vi "check_moving.vi"(8 "error in (no error)":errorcluster caption="错误输入（无错误）", 10 "用户事件":refnum<user-event>, 11 "MotorSystem 输入":refnum<class "MotorSystem.lvclass">) -> (0 "error out":errorcluster caption="错误输出", 3 "MotorSystem 输出":refnum<class "MotorSystem.lvclass">)   [LabVIEW 2016, in "MotionControl_UFO_3DOF.lvlib" / "MotorSystem.lvclass"]
uses:
  <userlib>/MotionControl_UFO_3DOF/MotorSystem/MotorSystem.lvclass
  <userlib>/MotionControl_UFO_3DOF/MotorSystem/MotorSystem.lvclass/MotorSystem.ctl
  <userlib>/MotionControl_UFO_3DOF/OneMotion/OneMotion.lvclass/OneMotion.ctl
  <userlib>/MotionControl_UFO_3DOF/StepMotor/StepMotor.lvclass/StepMotor.ctl
  <userlib>/UISimCanFunc_wrapper/ctl/Notice ID.ctl
  <userlib>/MotionControl_UFO_3DOF/StepMotor/StepMotor.lvclass
  <userlib>/MotionControl_UFO_3DOF/OneMotion/OneMotion.lvclass
  <userlib>/UISimCanFunc_wrapper/UISimCanFunc_wrapper.lvlib
panel:
  out "moving?":bool[](array[boolean])
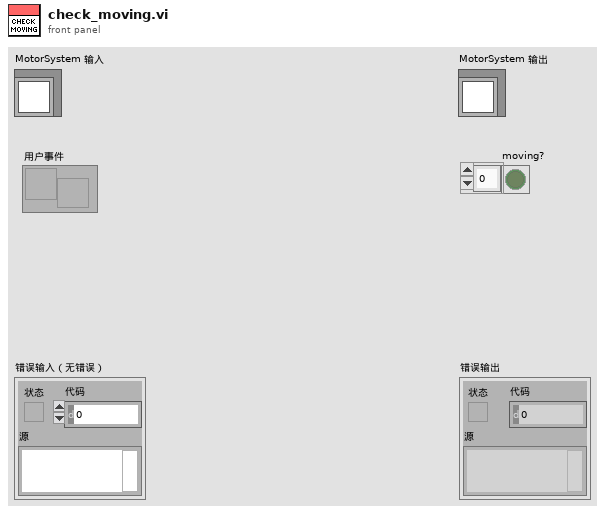
[diagram p1: front panel]
types:
  T1 = typedef "UISimCanFunc_wrapper.lvlib/Notice ID.ctl" = enum16{"S1 FALLING", "S1 RISING", "S2 FALLING", "S2 RISING", "S3 FALLING", "S3 RISING", "P4 DOUT LOW", "P4 DOUT HIGH", "MOVE DONE (OPEN LOOP)", "MOVE DONE (CLOSED LOOP)", "ORIGIN ARRIVED", "STALL NOTIFY", "MOVING", "STANDBY", "SET_TARGET_POS", "OTHERS"}
  T2 = typedef "MotionControl_UFO_3DOF.lvlib/MotorSystem.lvclass/MotionCluster.ctl" = cluster{"OneMotion.lvclass":refnum<class "OneMotion.lvclass">, "connected?":bool, "default enabled?":bool, "enabled?":bool}
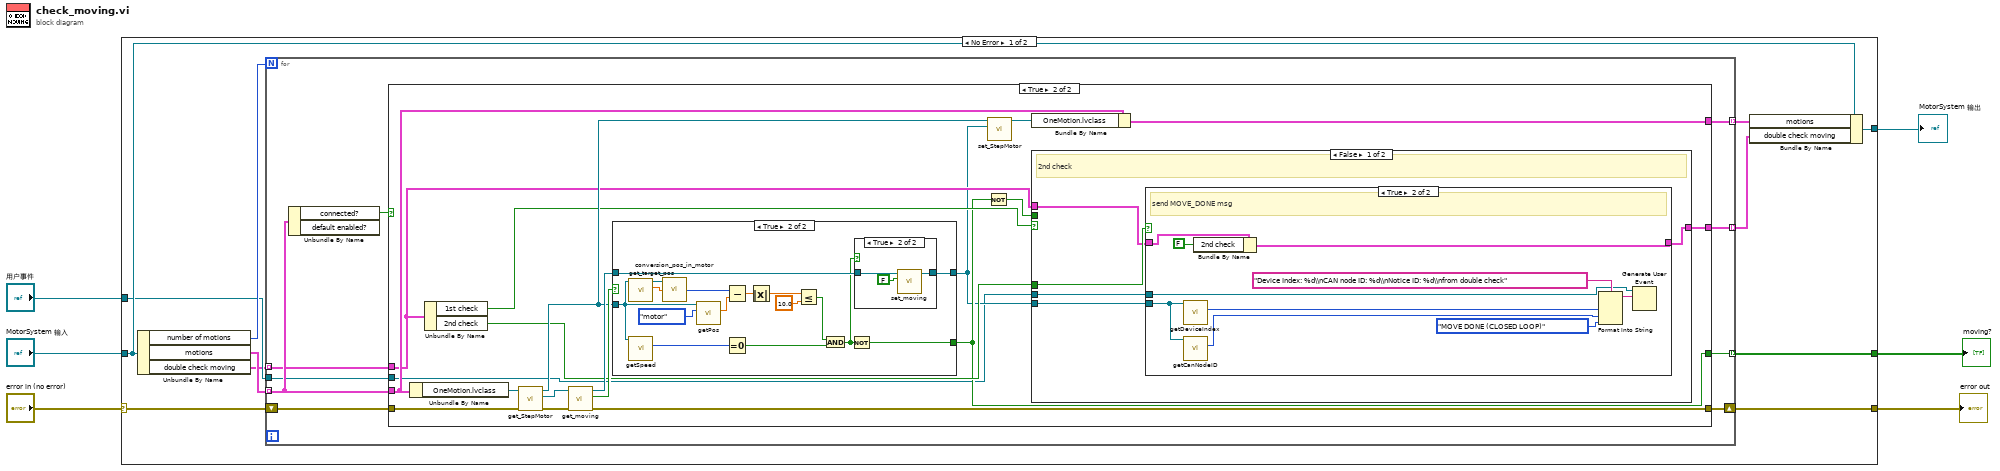
[diagram p0: block diagram]
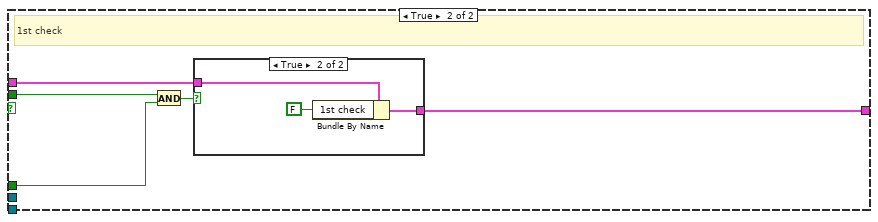
[diagram p4: hidden frame]
diagram:
  n1 = case shown="No Error" "error in (no error)" {
    tunnel: [w17 _] -> w4
    tunnel: "MotorSystem 输入" -> [w11 w96]
    tunnel: [w16 _] -> w3
    tunnel: [w13 w96] -> w5
    tunnel: "用户事件" -> [w10 _]
    selector: "error in (no error)" -> [w7 _]
    frame No Error {
      n2 = Unbundle By Name(w11) -> ("number of motions"=w15:i32, "motions"=w12:T2[], "double check moving"=w9:cluster{"1st check":bool, "2nd check":bool}[])
      n3 = for {
        N: w15 -> [_]
        tunnel: [w25] -> w16 mode=indexing
        tunnel: w12 -> [w23] mode=indexing
        shift-right: [w26] -> w17
        shift-left: w7 -> [w24]
        tunnel: [w21] -> w14 mode=indexing
        tunnel: w10 -> [w20]
        tunnel: w9 -> [w19] mode=indexing
        tunnel: [w18] -> w8 mode=indexing
        n4 = Unbundle By Name(w23) -> ("connected?"=w22:bool)  [unwired: 1 out]
        n5 = case shown="True" w22 {
          tunnel: [w29 w45] -> w26
          tunnel: [_ w34] -> w25
          tunnel: w23 -> [w28 w40]
          tunnel: w24 -> [w29 w44]
          tunnel: [w28 w38] -> w21
          tunnel: w20 -> [_ w30]
          tunnel: w19 -> [w27 w33]
          tunnel: [w27 w32] -> w18
          frame False {
          }
          frame True {
            n6 = Unbundle By Name(w40) -> ("OneMotion.lvclass"=w48:refnum<class "OneMotion.lvclass">)
            n7 = Unbundle By Name(w33) -> ("1st check"=w37:bool, "2nd check"=w35:bool)
            n8 = call <userlib>:"get_StepMotor.vi"("error in (no error)"=w44, "OneMotion输入"=w48) -> ("error out"=w46:errorcluster, "StepMotor.lvclass"=w47:refnum<class "StepMotor.lvclass">, "OneMotion输出"=w41:refnum<class "OneMotion.lvclass">)  [unwired: 7 in]
            n9 = call <userlib>:"get_moving.vi"("error in (no error)"=w46, "StepMotor输入"=w47) -> ("error out"=w45:errorcluster, "moving?"=w43:bool, "StepMotor输出"=w42:refnum<class "StepMotor.lvclass">)  [unwired: 7 in]
            n10 = case shown="True" w43 {
              selector: w43 -> [w74 _]
              tunnel: w41 -> [_ w81]
              tunnel: w42 -> [w75 w83]
              tunnel: [w75 w82] -> w31
              tunnel: [w74 w79] -> w34
              frame False {
              }
              frame True {
                n11 = call <userlib>:"get_target_pos.vi"("OneMotion输入"=w81) -> ("target pos"=w78:dbl, "OneMotion输出"=w91:refnum<class "OneMotion.lvclass">)  [unwired: 8 in, 1 out]
                n12 = call <userlib>:"getSpeed.vi"("OneMotion 输入"=w81) -> ("speed"=w76:i32)  [unwired: 8 in, 2 out]
                n13 = call <userlib>:"conversion_pos_in_motor.vi"("pos"=w78, "OneMotion 输入"=w91) -> ("pos in motor"=w89:i32)  [unwired: 1 in, 2 out]
                n14 = call <userlib>:"getPos.vi"("lab or motor"=enum16{"lab", "motor"}."motor", "OneMotion 输入"=w81) -> ("pos"=w77:dbl)  [unwired: 7 in, 2 out]
                n15 = Subtract(x=w89, y=w77) -> (x-y=w88:dbl)
                n16 = Equal To 0?(x=w76) -> (x = 0?=w85:bool)
                n17 = Absolute Value(x=w88) -> (abs(x)=w87:dbl)
                n18 = Less Or Equal?(x=w87, y=10.0) -> (x <= y?=w84:bool)
                n19 = And(x=w84, y=w85) -> (x .and. y?=w80:bool)
                n20 = Not(x=w80) -> (.not. x?=w79:bool)
                n21 = case shown="True" w80 {
                  tunnel: w83 -> [w92 w93]
                  tunnel: [w92 w94] -> w82
                  frame False {
                  }
                  frame True {
                    n22 = call <userlib>:"set_moving.vi"("moving?"=FALSE, "StepMotor输入"=w93) -> ("StepMotor输出"=w94:refnum<class "StepMotor.lvclass">)  [unwired: 8 in, 1 out]
                  }
                }
              }
            }
            n23 = Not(x=w34) -> (.not. x?=w36:bool)
            n24 = call <userlib>:"set_StepMotor.vi"("StepMotor.lvclass"=w31, "OneMotion输入"=w41) -> ("OneMotion输出"=w39:refnum<class "OneMotion.lvclass">)  [unwired: 8 in, 1 out]
            n25 = Bundle By Name(cluster=w40, "OneMotion.lvclass"=w39) -> (w38:T2)
            n26 = case shown="False" w37 {
              tunnel: w36 -> [_ w69]
              tunnel: w35 -> [w53 w68]
              tunnel: w33 -> [w52 w67]
              tunnel: [w51 w65] -> w32
              tunnel: w31 -> [w50 _]
              tunnel: w30 -> [w49 _]
              frame False {
                # "2nd check"
                n27 = case shown="True" w53 {
                  tunnel: w52 -> [w54 w64]
                  tunnel: [w54 w63] -> w51
                  tunnel: w50 -> [_ w56]
                  tunnel: w49 -> [_ w55]
                  frame False {
                  }
                  frame True {
                    # "send MOVE_DONE msg"
                    n28 = call-dynamic "getDeviceIndex.vi"("StepMotor输入"=w56) -> ("device index"=w58:u32)  [unwired: 8 in, 2 out]
                    n29 = call-dynamic "getCanNodeID.vi"("StepMotor输入"=w56) -> ("CAN node ID"=w59:u32)  [unwired: 8 in, 2 out]
                    n30 = Bundle By Name(cluster=w64, "2nd check"=FALSE) -> (w63:cluster{"1st check":bool, "2nd check":bool})
                    n31 = Format Into String(format string="Device Index: %d\\nCAN node ID: %d\\nNotice ID: %d\\nfrom double check", w58, w59, Notice_ID."MOVE DONE (CLOSED LOOP)" ("Notice ID")) -> (resulting string=w61:string)  [unwired: 2 in, 1 out]
                    n32 = Generate User Event(user event=w55, event data cluster=w61) -> ()  [unwired: 2 in, 2 out]
                  }
                }
              }
              frame True {
                # "1st check"
                n33 = And(x=w69, y=w68) -> (x .and. y?=w66:bool)
                n34 = case shown="True" w66 {
                  tunnel: w67 -> [w70 w73]
                  tunnel: [w70 w71] -> w65
                  frame False {
                  }
                  frame True {
                    n35 = Bundle By Name(cluster=w73, "1st check"=FALSE) -> (w71:cluster{"1st check":bool, "2nd check":bool})
                  }
                }
              }
            }
          }
        }
      }
      n36 = Bundle By Name(cluster=w11, "motions"=w14, "double check moving"=w8) -> (w13:refnum<class "MotorSystem.lvclass">)
    }
    frame Error {
    }
  }
  "error out" <- w4
  "MotorSystem 输出" <- w5
  "moving?" <- w3
